vi "Image_Save_Dequeue.vi"(0 "Data":T2={"L16 Linear Actuator"="", "XE 1000 Pump"="", "Camera1"="", "Camera2"="", "Img_Capt"=FALSE, "Actuator"=FALSE, "Pump"=FALSE, "Cam 1"=FALSE, "Cam 2"=FALSE, "Empty_Refill"=FALSE, "Crop"=FALSE, "Light intensity"=100, "Exposure Time"=1000.0, "Sample Name"="Test Sample", "Operator"="MRJ", "Calibration 1"=path "C:/Users/au540322/Desktop/IHS_Project/images/Debris/Debris_0/Debris_0_2019_06_01-23-32-49-686.PNG", "Calibration 2"=path "C:/Users/au540322/Desktop/IHS_Project/images/Debris/Debris_0/Debris_0_2019_06_01-23-32-49-686.PNG", "Framerate"=1, "Timeout Sample"=0, "Collection date"="MRJ", "Sample size threshold"=1, "Empty start"=1, "Command"="MRJ", "Station"="", "Species Name"="", "Other Notes"="", "Aperture"=enum."Item 0", "Image Process Queue Size"=500, "Image Save Queue Size"=500, "Overload threshold"=500, "Max Framerate"=100, "Rectangle 1"={"Left"=0, "Top"=0, "Right"=0, "Bottom"=0, "Rotation"=0.0}, "Rectangle 2"={"Left"=0, "Top"=0, "Right"=0, "Bottom"=0, "Rotation"=0.0}, "Detection Region %"=0.0, "Detect 1"=path "C:/Users/au540322/Desktop/IHS_Project/images/Debris/Debris_0/Debris_0_2019_06_01-23-32-49-686.PNG", "Detect 2"=path "C:/Users/au540322/Desktop/IHS_Project/images/Debris/Debris_0/Debris_0_2019_06_01-23-32-49-686.PNG", "Max large object threshold"=0, "Open(T)/Close(F)"=FALSE, "Img_Capt Begin"=FALSE, "Dispense Speed"=100, "Flush Size"=100, "Location"="Station", "Latitude"="Station", "Longitude"="Station", "Determiner"="Station", "Sex"="Station", "Camera1_Img"=refnum, "Camera2_Img"=refnum, "Img1_Orig_Disp"=refnum, "Img2_Orig_Disp"=refnum, "Img1_Orig_RGB"=refnum, "Img2_Orig_RGB"=refnum, "Blue_Plane_Extract"=refnum, "Subtracted_Plane"=refnum, "Img1_Binary"=refnum, "Img2_Binary"=refnum, "Crop_Mask"=refnum, "Img1_Save"=refnum, "Img2_Save"=refnum, "Img1_Cali_Full"=refnum, "Img2_Cali_Full"=refnum, "Img1_Cali_Detect"=refnum, "Img2_Cali_Detect"=refnum, "Cam 1 queue"=refnum, "Cam 2 queue"=refnum, "Cam 1 - save queue"=refnum, "Cam 2 - save queue"=refnum} {"Flush Size" min=1; "Dispense Speed" min=1; "Rectangle 2"."Rotation" format="%.2f"; "Rectangle 2"."Left" scale=0.0..1024.0; "Rectangle 2"."Right" scale=0.0..1024.0; "Rectangle 1"."Rotation" format="%.2f"; "Rectangle 1"."Left" scale=0.0..1024.0; "Rectangle 1"."Right" scale=0.0..1024.0; "Max Framerate" min=1; "Overload threshold" min=1; "Image Save Queue Size" min=1; "Image Process Queue Size" min=1; "Empty start" min=1; "Sample size threshold" min=1; "Framerate" min=1; "Light intensity" scale=0.0..100.0}, 5 "Camera":T5, 7 "Old":i32, 9 "Other":i32, 11 "Queue active":bool) -> (3 "timed out?":bool, 4 "# elements in queue":i32, 6 "State out":i32, 8 "Image Save 1":T1, 10 "Image Save 2":T1, 14 "Sample Data":dbl[](array[numeric]), 15 "Last image":bool)   [LabVIEW 2020]
uses:
  Camera_ID.ctl
  controls/Data.ctl
  <vilib>/userDefined/High Color/IMAQdx.ctl
  <vilib>/vision/Image Controls.llb/IMAQ Image.ctl
panel:
  out "error out":errorcluster
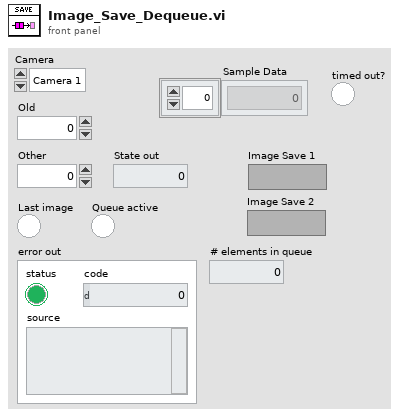
[diagram p1: front panel]
types:
  T1 = typedef "IMAQ Image.ctl" = refnum<image>
  T2 = typedef "Data.ctl" = cluster{"L16 Linear Actuator":refnum<visa-resource-name>, "XE 1000 Pump":refnum<visa-resource-name>, "Camera1":T3, "Camera2":T3, "Img_Capt":bool, "Actuator":bool, "Pump":bool, "Cam 1":bool, "Cam 2":bool, "Empty_Refill":bool, "Crop":bool, "Light intensity":i32, "Exposure Time":dbl, "Sample Name":string, "Operator":string, "Calibration 1":path, "Calibration 2":path, "Framerate":i32, "Timeout Sample":i32, "Collection date":string, "Sample size threshold":i32, "Empty start":u32, "Command":string, "Station":string, "Species Name":string, "Other Notes":string, "Aperture":enum32{"Item 0", "Item 1", "Item 2", "Item 3"}, "Image Process Queue Size":i32, "Image Save Queue Size":i32, "Overload threshold":i32, "Max Framerate":i32, "Rectangle 1":T4, "Rectangle 2":T4, "Detection Region %":dbl, "Detect 1":path, "Detect 2":path, "Max large object threshold":i32, "Open(T)/Close(F)":bool, "Img_Capt Begin":bool, "Dispense Speed":i32, "Flush Size":i32, "Location":string, "Latitude":string, "Longitude":string, "Determiner":string, "Sex":string, "Camera1_Img":T1, "Camera2_Img":T1, "Img1_Orig_Disp":T1, "Img2_Orig_Disp":T1, "Img1_Orig_RGB":T1, "Img2_Orig_RGB":T1, "Blue_Plane_Extract":T1, "Subtracted_Plane":T1, "Img1_Binary":T1, "Img2_Binary":T1, "Crop_Mask":T1, "Img1_Save":T1, "Img2_Save":T1, "Img1_Cali_Full":T1, "Img2_Cali_Full":T1, "Img1_Cali_Detect":T1, "Img2_Cali_Detect":T1, "Cam 1 queue":refnum<queue>, "Cam 2 queue":refnum<queue>, "Cam 1 - save queue":refnum<queue>, "Cam 2 - save queue":refnum<queue>}
  T3 = typedef "IMAQdx.ctl" = refnum<k21>
  T4 = typedef "IMAQ Rectangle" = cluster{"Left":i32, "Top":i32, "Right":i32, "Bottom":i32, "Rotation":dbl}
  T5 = typedef "Camera_ID.ctl" = enum16{"Camera 1", "Camera 2"}
  T6 = cluster{"Timestamp":string, "Image Pixels (U32)":u32[][], "Prev. sample":i32, "Sample Data":dbl[], "output cluster":cluster{"Global Rectangle":i32[], "Contours":cluster{"ID":enum32{"External", "Internal"}, "Type":u32, "Coordinates":i32[]}[]}}
  T7 = cluster{"Global Rectangle":i32[], "Contours":cluster{"ID":enum32{"External", "Internal"}, "Type":u32, "Coordinates":i32[]}[]}
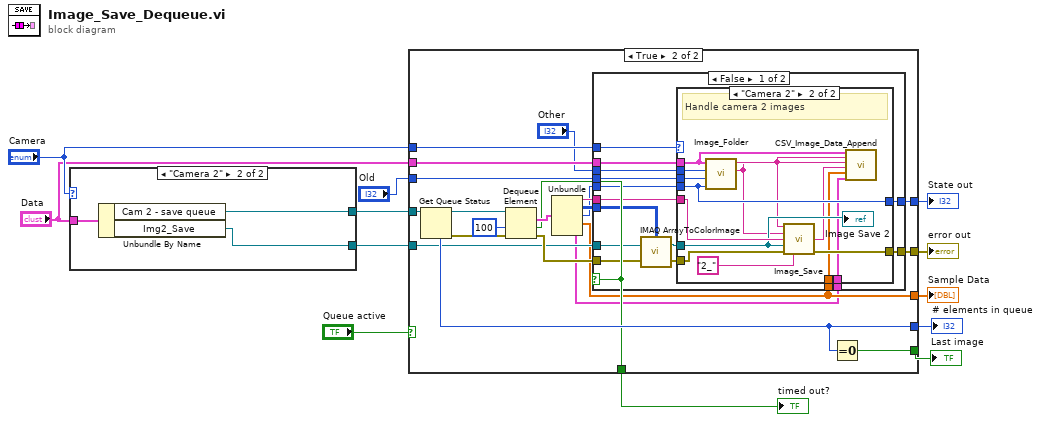
[diagram p0: block diagram]
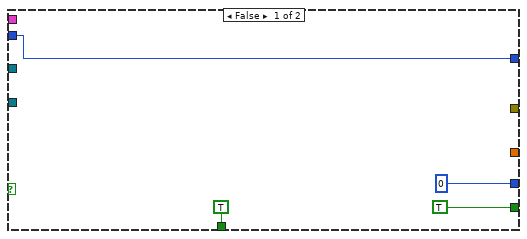
[diagram p2: hidden frame]
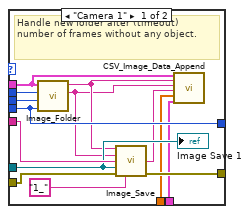
[diagram p3: hidden frame]
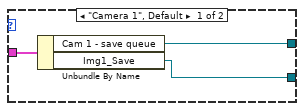
[diagram p5: hidden frame]
diagram:
  n1 = case shown="\"Camera 2\"" "Camera" {
    tunnel: [w14 w18] -> w11
    tunnel: "Data" -> [w15 w17]
    tunnel: [w13 w16] -> w1
    frame "Camera 1", Default {
      n2 = Unbundle By Name(w15) -> ("Cam 1 - save queue"=w14:refnum<queue>, "Img1_Save"=w13:T1)
    }
    frame "Camera 2" {
      n3 = Unbundle By Name(w17) -> ("Cam 2 - save queue"=w18:refnum<queue>, "Img2_Save"=w16:T1)
    }
  }
  n4 = case shown="True" "Queue active" {
    tunnel: "Camera" -> [_ w43]
    tunnel: w11 -> [_ w39]
    tunnel: "Data" -> [_ w38]
    tunnel: [0 ("# elements in queue") w37] -> w8
    tunnel: [TRUE w36] -> w7
    tunnel: [_ w35] -> w6
    tunnel: [w20 w30] -> w5
    tunnel: "Old" -> [w20 w29]
    tunnel: [_ w24] -> w3
    tunnel: [TRUE ("timed out?") w27] -> w2
    tunnel: w1 -> [_ w25]
    frame False {
    }
    frame True {
      n5 = Get Queue Status(queue=w39) -> (queue out=w40:refnum<queue>, error out=w33:errorcluster, # elements in queue=w37:i32)  [unwired: 2 in, 5 out]
      n6 = Dequeue Element(queue=w40, timeout in ms (-1)=100, error in (no error)=w33) -> (element=w42:T6, timed out?=w27:bool, error out=w26:errorcluster)  [unwired: 1 out]
      n7 = Unbundle(w42) -> ("Timestamp"=w34:string, "Image Pixels (U32)"=w41:u32[][], "Prev. sample"=w32:i32, "Sample Data"=w24:dbl[], "output cluster"=w23:T7)
      n8 = case shown="False" w27 {
        tunnel: w43 -> [w58 _]
        tunnel: w41 -> [w46 _]
        tunnel: w38 -> [w57 _]
        tunnel: [w56 w87] -> w35
        tunnel: w34 -> [w55 _]
        tunnel: w32 -> [w54 _]
        tunnel: "Other" -> [w53 _]
        tunnel: [w52 w88] -> w30
        tunnel: w29 -> [w51 w88]
        tunnel: w26 -> [w47 w87]
        tunnel: w25 -> [w50 _]
        tunnel: w24 -> [w45 _]
        tunnel: w23 -> [w44 _]
        frame False {
          n9 = call "IMAQ ArrayToColorImage"("Image Pixels (U32)"=w46, "Image"=w50, "error in (no error)"=w47) -> ("Image Out"=w49:T1, "error out"=w48:errorcluster)  [unwired: 2 in]
          n10 = case shown="\"Camera 2\"" w58 {
            tunnel: [w72 w86] -> w56
            tunnel: w49 -> [w65 w79]
            tunnel: w57 -> [w64 w78]
            tunnel: w55 -> [w70 w84]
            tunnel: w48 -> [w69 w83]
            tunnel: w54 -> [w66 w80]
            tunnel: w51 -> [w68 w82]
            tunnel: w53 -> [w67 w81]
            tunnel: [w66 w80] -> w52
            tunnel: w45 -> [w60 w74]
            tunnel: w44 -> [w59 w73]
            frame "Camera 1" {
              # "Handle new folder after (timeout) number of frames without any object."
              n11 = call "Image_Folder.vi"("New"=w66, "Old"=w68, "Other"=w67, "input cluster"=w64) -> ("Subfolder Name"=w62:string, "Subfolder Path"=w63:string)  [unwired: 6 in]
              n12 = call "Image_Save.vi"("Subfolder path"=w63, "Subfolder Name"=w62, "Timestamp"=w70, "Image in"=w65, "error in"=w69, "Camera"="1_" ("Camera image prefix")) -> ("Image Name"=w61:string, "error out"=w72:errorcluster)  [unwired: 6 in, 2 out]
              n13 = call "CSV_Image_Data_Append.vi"("input cluster"=w64, "Image path"=w63, "Sample Name"=w62, "Image Name"=w61, "Sample Data"=w60, "ROI Descriptor"=w59) -> ()  [unwired: 14 in]
              "Image Save 1" <- w65
            }
            frame "Camera 2" {
              # "Handle camera 2 images"
              n14 = call "Image_Folder.vi"("New"=w80, "Old"=w82, "Other"=w81, "input cluster"=w78) -> ("Subfolder Name"=w76:string, "Subfolder Path"=w77:string)  [unwired: 6 in]
              n15 = call "Image_Save.vi"("Subfolder path"=w77, "Subfolder Name"=w76, "Timestamp"=w84, "Image in"=w79, "error in"=w83, "Camera"="2_" ("Camera image prefix")) -> ("Image Name"=w75:string, "error out"=w86:errorcluster)  [unwired: 6 in, 2 out]
              n16 = call "CSV_Image_Data_Append.vi"("input cluster"=w78, "Image path"=w77, "Sample Name"=w76, "Image Name"=w75, "Sample Data"=w74, "ROI Descriptor"=w73) -> ()  [unwired: 14 in]
              "Image Save 2" <- w79
            }
          }
        }
        frame True {
        }
      }
      n17 = Equal To 0?(x=w37) -> (x = 0?=w36:bool)
    }
  }
  "# elements in queue" <- w8
  "Last image" <- w7
  "error out" <- w6
  "State out" <- w5
  "Sample Data" <- w3
  "timed out?" <- w2
